vi "Equals.vi"(10 "String":string, 11 "Section Name in":refnum<class "Section Name.lvclass">) -> (2 "Equal?":bool, 3 "Section Name out":refnum<class "Section Name.lvclass">)   [LabVIEW 2024, in "Electronic Datasheet.lvlib" / "Section Name.lvclass"]
uses:
  Section Name.lvclass
  Section Name.lvclass/Section Name.ctl
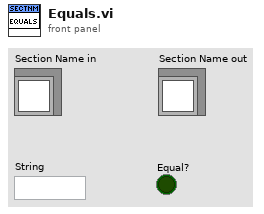
[diagram p1: front panel]
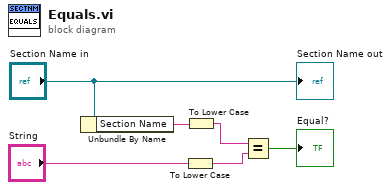
[diagram p0: block diagram]
diagram:
  n1 = Unbundle By Name("Section Name in") -> ("Section Name"=w5:string)
  n2 = To Lower Case(string="String") -> (all lower case string=w2:string)
  n3 = To Lower Case(string=w5) -> (all lower case string=w3:string)
  n4 = Equal?(x=w3, y=w2) -> (x = y?=→"Equal?":bool)
  "Section Name out" <- "Section Name in"
